vi "Stop Receiving.vi"(8 "error in (no error)":errorcluster, 11 "Vision Receiver in":refnum<class "Vision Receiver.lvclass">) -> (0 "error out":errorcluster, 3 "Vision Receiver out":refnum<class "Vision Receiver.lvclass">)   [LabVIEW 2022 SP3, in "Vision Receiver.lvlib" / "Vision Receiver.lvclass"]
uses:
  Vision Receiver.lvclass
  Vision Receiver.lvclass/Vision Receiver.ctl
  UDP Reader/UDP Reader Messages/Halt Msg/Halt Msg.lvclass
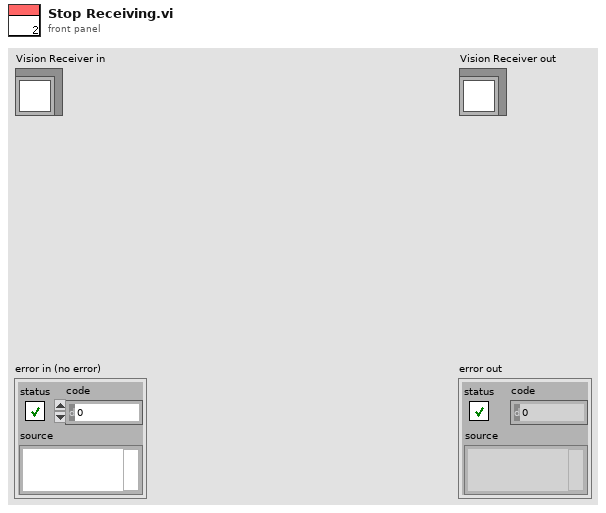
[diagram p1: front panel]
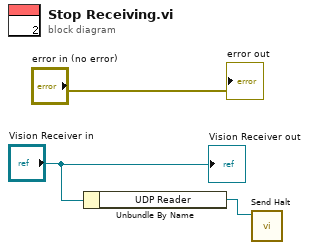
[diagram p0: block diagram]
diagram:
  n1 = Unbundle By Name("Vision Receiver in") -> ("UDP Reader"=w2:refnum<class "Message Enqueuer.lvclass">)
  n2 = call "Send Halt.vi"("Message Enqueuer"=w2) -> ()  [unwired: 9 in, 2 out]
  "error out" <- "error in (no error)"
  "Vision Receiver out" <- "Vision Receiver in"
